vi "Write Language File.vi"   [LabVIEW 2018]
uses:
  <vilib>/Utility/file.llb/Write Delimited Spreadsheet (string).vi
panel:
  # "This VI creates the language file used by the coffee maker."
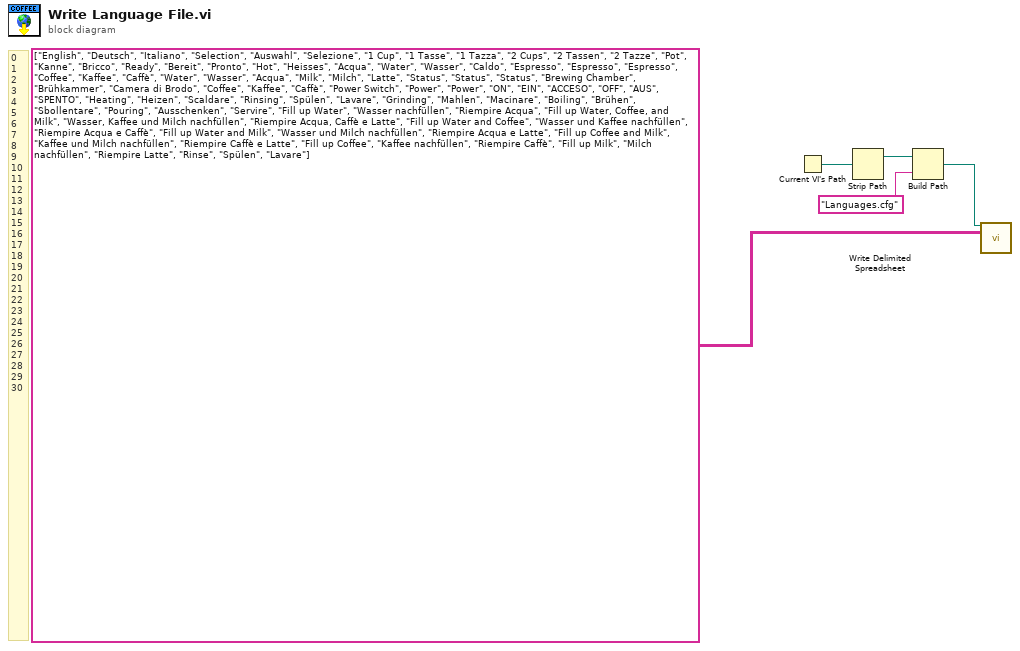
[diagram p0: block diagram]
diagram:
  # "0\n1\n2\n3\n4\n5\n6\n7\n8\n9\n10\n11\n12\n13\n14\n15\n16\n17\n18\n19\n20\n21\n22\n23\n24\n25\n26\n27\n28\n29\n30"
  n1 = Current VI's Path() -> (path=w4:path)
  n2 = Strip Path(path=w4) -> (stripped path=w3:path)  [unwired: 1 out]
  n3 = Build Path(base path=w3, name or relative path="Languages.cfg") -> (appended path=w1:path)
  n4 = call-poly <vilib>:"Write Delimited Spreadsheet.vi"("file path (dialog if empty)"=w1, "2D data"=string[][] [["English", "Deutsch", "Italiano"], ["Selection", "Auswahl", "Selezione"], ["1 Cup", "1 Tasse", "1 Tazza"], ["2 Cups", "2 Tassen", "2 Tazze"], ["Pot", "Kanne", "Bricco"], ["Ready", "Bereit", "Pronto"], ["Hot", "Heisses", "Acqua"], ["Water", "Wasser", "Caldo"], ["Espresso", "Espresso", "Espresso"], ["Coffee", "Kaffee", "Caffè"], ["Water", "Wasser", "Acqua"], ["Milk", "Milch", "Latte"], ["Status", "Status", "Status"], ["Brewing Chamber", "Brühkammer", "Camera di Brodo"], ["Coffee", "Kaffee", "Caffè"], ["Power Switch", "Power", "Power"], ["ON", "EIN", "ACCESO"], ["OFF", "AUS", "SPENTO"], ["Heating", "Heizen", "Scaldare"], ["Rinsing", "Spülen", "Lavare"], ["Grinding", "Mahlen", "Macinare"], ["Boiling", "Brühen", "Sbollentare"], ["Pouring", "Ausschenken", "Servire"], ["Fill up Water", "Wasser nachfüllen", "Riempire Acqua"], ["Fill up Water, Coffee, and Milk", "Wasser, Kaffee und Milch nachfüllen", "Riempire Acqua, Caffè e Latte"], ["Fill up Water and Coffee", "Wasser und Kaffee nachfüllen", "Riempire Acqua e Caffè"], ["Fill up Water and Milk", "Wasser und Milch nachfüllen", "Riempire Acqua e Latte"], ["Fill up Coffee and Milk", "Kaffee und Milch nachfüllen", "Riempire Caffè e Latte"], ["Fill up Coffee", "Kaffee nachfüllen", "Riempire Caffè"], ["Fill up Milk", "Milch nachfüllen", "Riempire Latte"], ["Rinse", "Spülen", "Lavare"]]) -> ()  [unwired: 12 in, 2 out]
